vi "SetParam.vi"(8 "error in (no error)":errorcluster caption="entrée d'erreur (pas d'erreur)", 10 "SkewedChi2Sampler":T1={"skewedness"=1.0, "n_components"=100, "random_state"=-1} {"random_state" min=-1}, 11 "SkewedChi2Sampler.lvclass":refnum<class "SkewedChi2Sampler.lvclass">) -> (0 "error out":errorcluster caption="sortie d'erreur", 3 "SkewedChi2Sampler.lvclass":refnum<class "SkewedChi2Sampler.lvclass">)   [LabVIEW 2020, in "SkewedChi2Sampler.lvclass"]
doc: "Set Parameters"
uses:
  SkewedChi2Sampler.lvclass
  SkewedChi2Sampler.lvclass/SkewedChi2Sampler.ctl
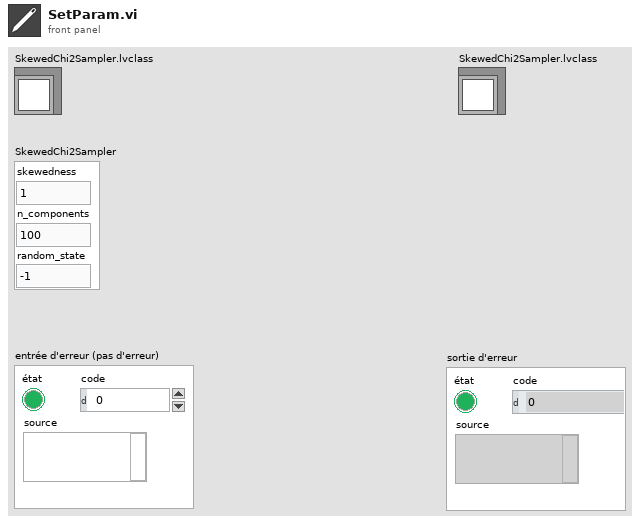
[diagram p1: front panel]
types:
  T1 = cluster{"skewedness":dbl, "n_components":i32, "random_state":i32}
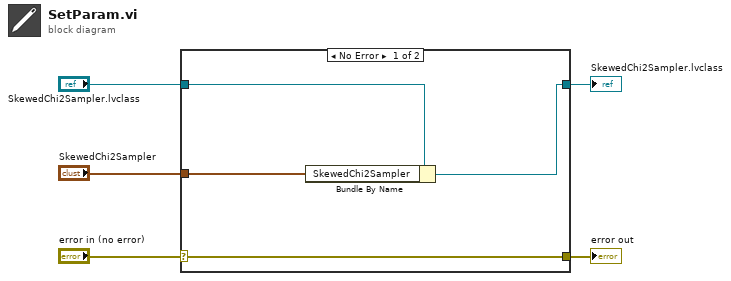
[diagram p0: block diagram]
diagram:
  n1 = case shown="No Error" "error in (no error)" {
    selector: "error in (no error)" -> [w9 w10]
    tunnel: [w9 w10] -> w4
    tunnel: [w7 w11] -> w2
    tunnel: "SkewedChi2Sampler.lvclass" -> [w8 w11]
    tunnel: "SkewedChi2Sampler" -> [w6 _]
    frame No Error {
      n2 = Bundle By Name(cluster=w8, "SkewedChi2Sampler"=w6) -> (w7:refnum<class "SkewedChi2Sampler.lvclass">)
    }
    frame Error {
    }
  }
  "error out" <- w4
  "SkewedChi2Sampler.lvclass" <- w2
